vi "_Main_LookOnly_DAC2022.vi"() -> ()   [LabVIEW 2017]
uses:
  <vilib>/Instr/_visa.llb/VISA Configure Serial Port (Instr).vi
panel:
  out "16bit integer":i16
  in  "DAC 1, V":dbl min=-50.0 max=50.0 format="%#_5g"
  in  "Stop Button":bool
  in  "Start Button":bool
  in  "COM port":refnum<visa-resource-name>
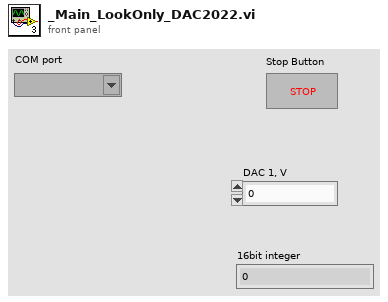
[diagram p1: front panel]
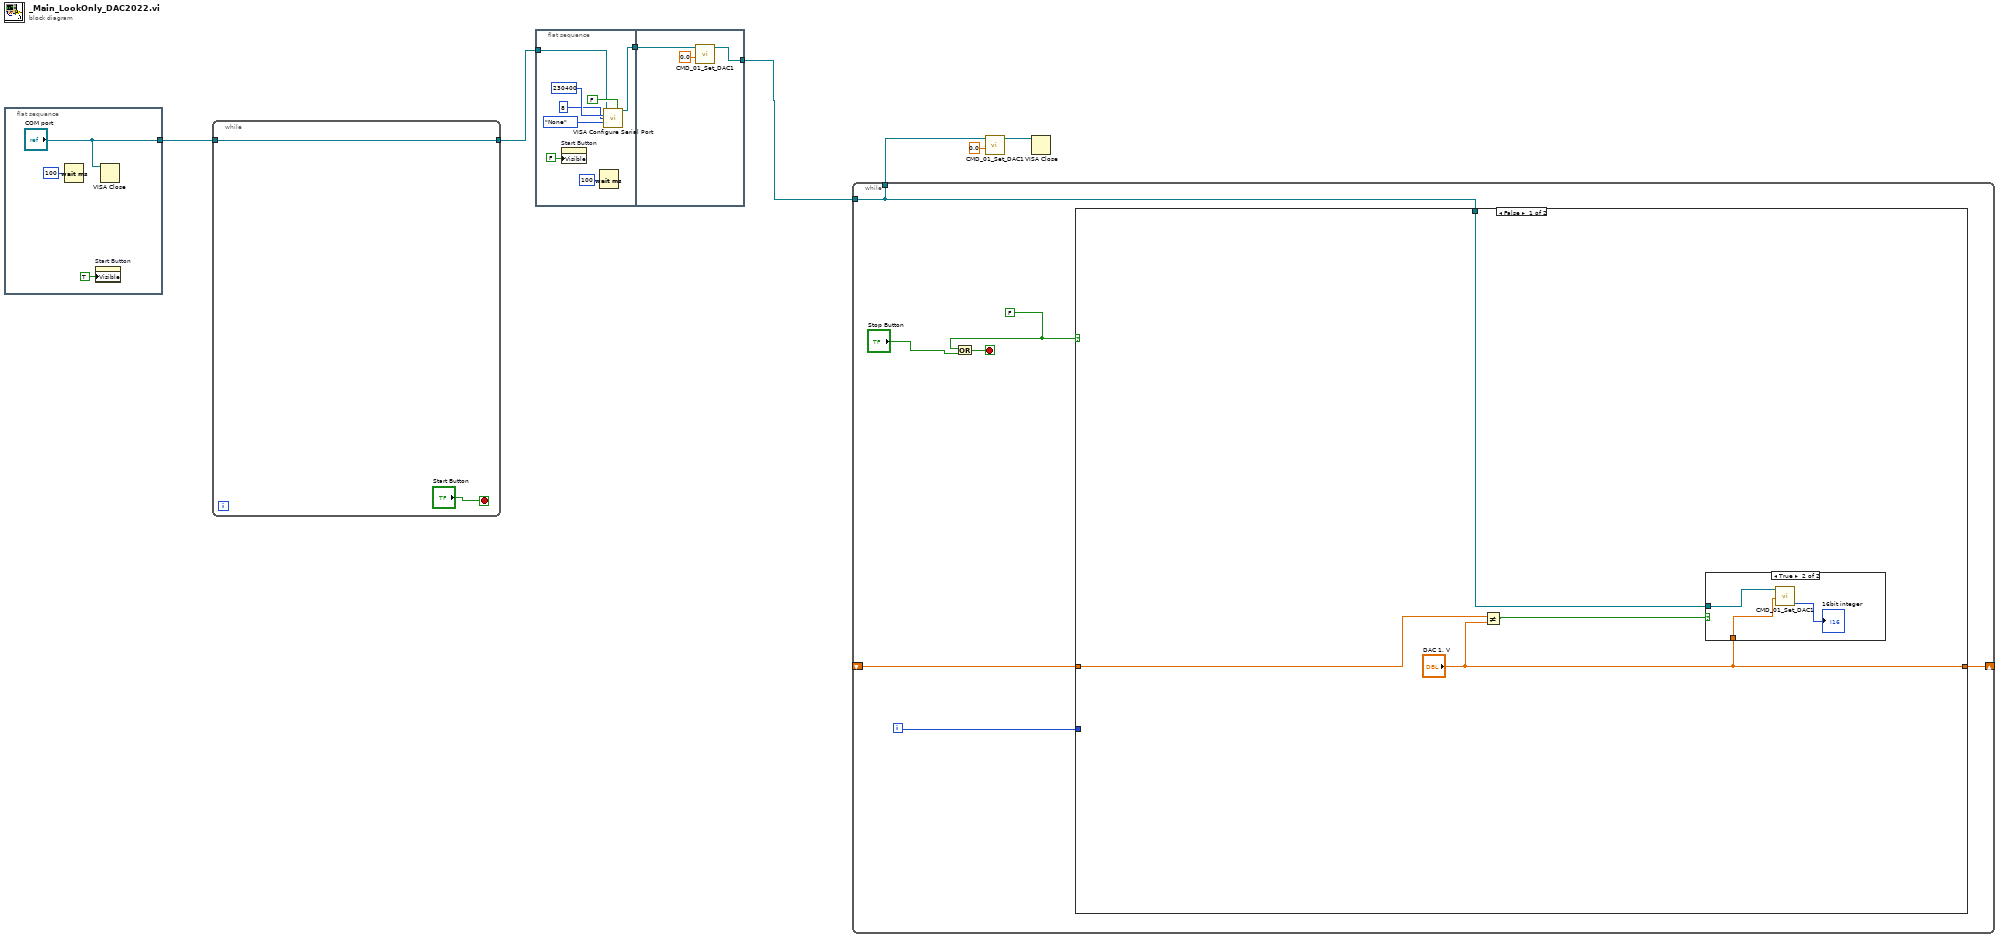
[diagram p0: block diagram]
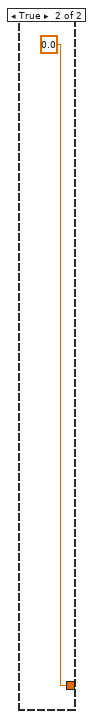
[diagram p3: hidden frame]
diagram:
  n1 = flat-sequence {
    tunnel: ["COM port"] -> w7
    frame #0 {
      n2 = Wait (ms)(milliseconds to wait=u32 100) -> ()  [unwired: 1 out]
      n3 = property on="Start Button" class="Bool"("Visible"=TRUE) -> ()  [unwired: 2 in, 2 out]
      n4 = VISA Close(VISA resource name="COM port") -> ()  [unwired: 1 in, 1 out]
    }
  }
  n5 = while {
    tunnel: w7 -> [w11]
    tunnel: [w11] -> w6
    stop <- "Start Button" stop-if-true
  }
  n6 = flat-sequence {
    tunnel: w6 -> [w16]
    tunnel: [w15] -> w2
    tunnel: [w23] -> w1
    tunnel: w2 -> [w22]
    frame #0 {
      n7 = property on="Start Button" class="Bool"("Visible"=FALSE) -> ()  [unwired: 2 in, 2 out]
      n8 = Wait (ms)(milliseconds to wait=u32 100) -> ()  [unwired: 1 out]
      n9 = call-poly "VISA Configure Serial Port"("VISA resource name"=w16, "Enable Termination\nChar (T)"=FALSE ("Enable Termination\nChar (T)"), "baud rate (9600)"=u32 230400, "data bits (8)"=u16 8, "parity (0:none)"=enum16{"None", "Odd", "Even", "Mark", "Space"}."None") -> ("VISA resource name out"=w15:refnum<visa-resource-name>)  [unwired: 9 in, 1 out]
    }
    frame #1 {
      n10 = call "CMD_01_Set_DAC1.vi"("Input, V"=0.0, "VISA resource name"=w22) -> ("VISA resource name out"=w23:refnum<visa-resource-name>)  [unwired: 8 in, 1 out]
    }
  }
  n11 = while {
    tunnel: w1 -> [w28]
    tunnel: [w28] -> w5
    shift-right: [w26] -> _
    shift-left: _ -> [w25]
    i -> [w29]
    stop <- w30 stop-if-true
    w24 = FALSE ("x")
    n12 = Or(x=w24, y="Stop Button") -> (x .or. y?=w30:bool)
    n13 = case shown="False" w24 {
      tunnel: w29 -> [_ _]
      tunnel: w28 -> [w33 _]
      tunnel: ["DAC 1, V" 0.0 ("DAC 1, V")] -> w26
      tunnel: w25 -> [w34 _]
      frame False {
        n14 = Not Equal?(x=w34, y="DAC 1, V") -> (x != y?=w31:bool)
        n15 = case shown="True" w31 {
          tunnel: "DAC 1, V" -> [_ w36]
          tunnel: w33 -> [_ w37]
          frame False {
          }
          frame True {
            n16 = call "CMD_01_Set_DAC1.vi"("Input, V"=w36, "VISA resource name"=w37) -> ("16bit integer"=→"16bit integer":i16)  [unwired: 8 in, 1 out]
          }
        }
      }
      frame True {
      }
    }
  }
  n17 = call "CMD_01_Set_DAC1.vi"("Input, V"=0.0, "VISA resource name"=w5) -> ("VISA resource name out"=w3:refnum<visa-resource-name>)  [unwired: 8 in, 1 out]
  n18 = VISA Close(VISA resource name=w3) -> ()  [unwired: 1 in, 1 out]
